vi "getListboxReference.vi"(11 "Setting in":refnum<class "Setting.lvclass">) -> (2 "ListboxReference":refnum<vi>, 3 "Setting out":refnum<class "Setting.lvclass">)   [LabVIEW 2020, in "Settings.lvlib" / "Setting.lvclass"]
uses:
  Setting.lvclass
  Setting.lvclass/Setting.ctl
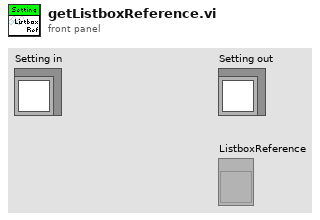
[diagram p1: front panel]
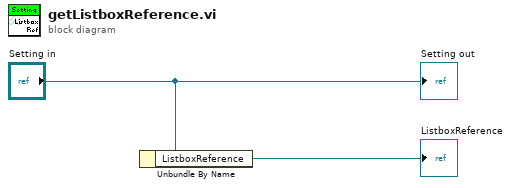
[diagram p0: block diagram]
diagram:
  n1 = Unbundle By Name("Setting in") -> ("ListboxReference"=→"ListboxReference":refnum<vi>)
  "Setting out" <- "Setting in"
